vi "openCommunication.vi"(8 "error in (no error)":errorcluster, 11 "PLC in":refnum<class "PLC.lvclass">) -> (0 "error out":errorcluster, 3 "PLC out":refnum<class "PLC.lvclass">)   [LabVIEW 2020, in "PLC.lvclass"]
uses:
  PLC.lvclass
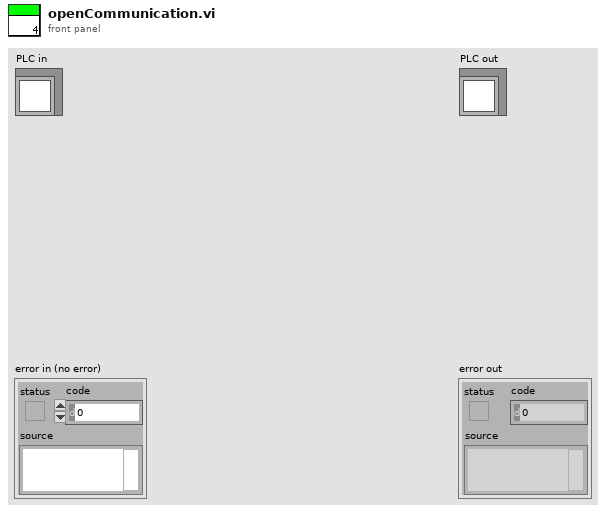
[diagram p1: front panel]
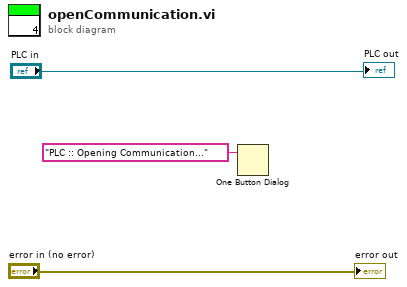
[diagram p0: block diagram]
diagram:
  n1 = One Button Dialog(message="PLC :: Opening Communication...") -> ()  [unwired: 1 in, 1 out]
  "error out" <- "error in (no error)"
  "PLC out" <- "PLC in"
